vi "In Place Read Scalar SGL.vi"(8 "error in (no error)":errorcluster, 10 "value in":sgl format="%#_13g", 11 "pointer in":u64) -> (0 "error out":errorcluster, 2 "value out":sgl, 3 "pointer out":u64)   [LabVIEW 2013, in "Linux RT IPC.Shared Memory.lvlib"]
uses:
  Linux RT IPC.Shared Memory.lvlib
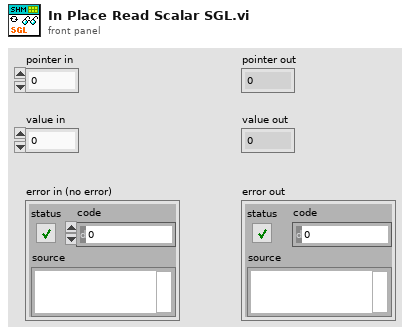
[diagram p1: front panel]
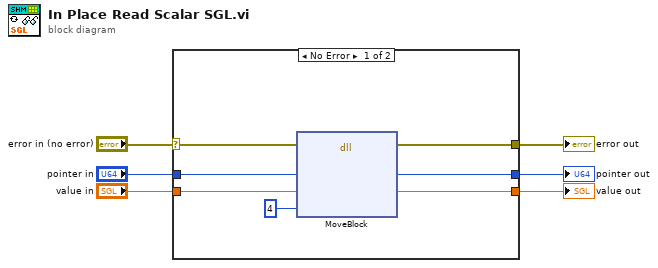
[diagram p0: block diagram]
diagram:
  n1 = case shown="No Error" "error in (no error)" {
    selector: "error in (no error)" -> [w12 w15]
    tunnel: [w11 w15] -> w6
    tunnel: "pointer in" -> [w10 w14]
    tunnel: [w9 w14] -> w3
    tunnel: [w8 _] -> w2
    tunnel: "value in" -> [w7 _]
    frame No Error {
      n2 = dll-call lib="LabVIEW" fn="MoveBlock"(error in=w12, "pointer"=w10, "data"=w7, "size"=u64 4) -> (error out=w11:errorcluster, "pointer"=w9:u64, "data"=w8:sgl)  [unwired: 4 in, 1 out]
    }
    frame Error {
    }
  }
  "error out" <- w6
  "pointer out" <- w3
  "value out" <- w2
